vi "OW Write Bytes.vi"(7 "WriteDataLen":u32, 9 "pWriteData":u8[](array[numeric])=array[4097 elements], 10 "ChannelMask":u32, 11 "DevHandle":i32) -> (1 "pWriteData out":u8[](array[numeric]), 3 "function return":i32)   [LabVIEW 2010, in "usb2ow.lvlib"]
doc: "int WINAPI OW_WriteBytes(int DevHandle, unsigned int ChannelMask,unsigned char *pWriteData,unsigned int WriteDataLen);"
uses:
  usb2ow.lvlib
  USB2XXX/trunk/USB2XXX/USB2XXX/vs2010/Release/USB2XXX.dll
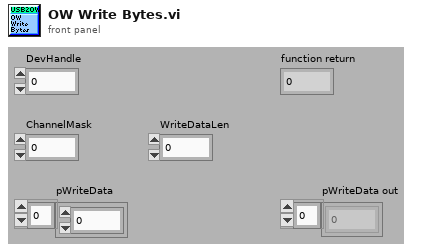
[diagram p1: front panel]
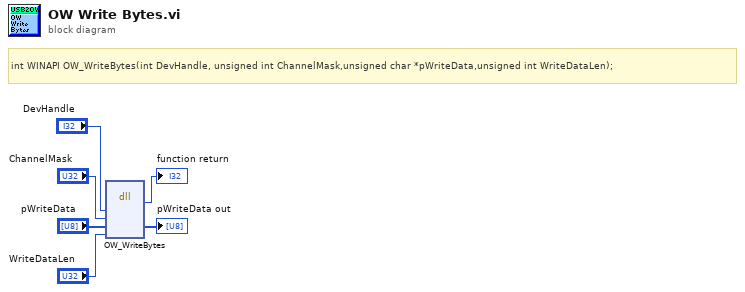
[diagram p0: block diagram]
diagram:
  # "int WINAPI OW_WriteBytes(int DevHandle, unsigned int ChannelMask,unsigned char *pWriteData,unsigned int WriteDataLen);"
  n1 = dll-call lib="E:/OtherWork/STM32/USB2XXX/trunk/USB2XXX/USB2XXX/vs2010/Release/USB2XXX.*" fn="OW_WriteBytes"("DevHandle"="DevHandle", "ChannelMask"="ChannelMask", "pWriteData"="pWriteData", "WriteDataLen"="WriteDataLen") -> (→"function return":i32, "pWriteData"=→"pWriteData out":u8[])  [unwired: 6 in, 2 out]
